vi "Get Strings from Ref.vi"(8 "error in (no error)":errorcluster, 9 "Label Prefix":string, 10 "GObj Refnum in":refnum<vi>, 11 "ArrayConstant in":refnum<class "ArrayControl.lvclass">) -> (0 "error out":errorcluster, 1 "Valid?":bool, 2 "GObj Refnum out":refnum<vi>, 3 "ArrayConstant out":refnum<class "ArrayControl.lvclass">, 4 "GObj Name":string)   [LabVIEW 2013, in "SET Project Data.lvlib" / "ArrayControl.lvclass"]
uses:
  ArrayControl.lvclass
  Control/Control.lvclass
  GObject/GObject.lvclass/GObject.ctl
  GObject/Write UID.vi
  GObject/GObject.lvclass
  SET Project Data.lvlib
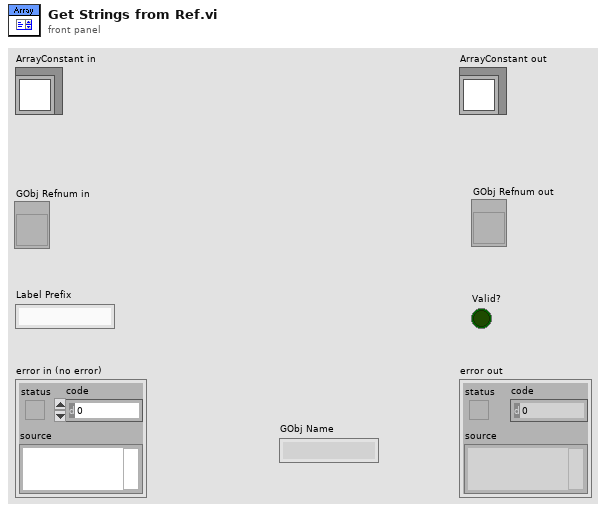
[diagram p1: front panel]
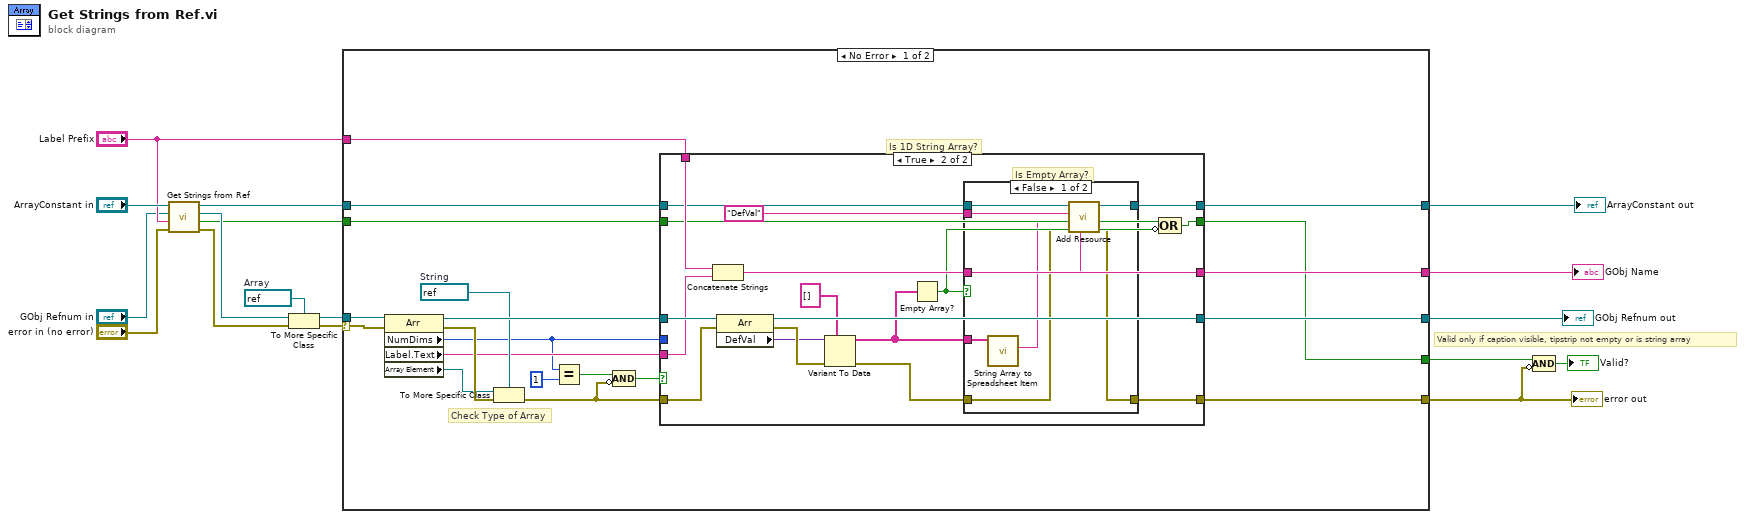
[diagram p0: block diagram]
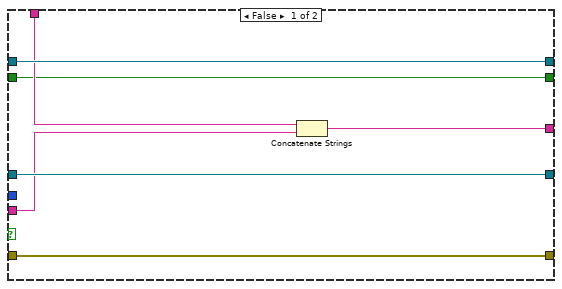
[diagram p2: hidden frame]
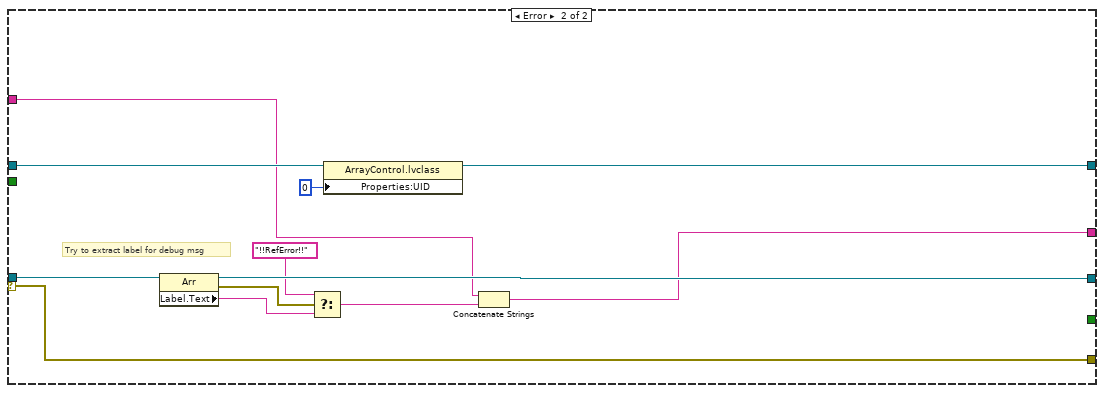
[diagram p4: hidden frame]
diagram:
  w9 = refnum<vi> refnum  # Array
  # "Valid only if caption visible, tipstrip not empty or is string array"
  n1 = call-parent "Get Strings from Ref.vi"("error in (no error)"="error in (no error)", "Label Prefix"="Label Prefix", "GObj Refnum in"="GObj Refnum in", "Control in"="ArrayConstant in") -> ("error out"=w5:errorcluster, "Valid?"=w1:bool, "GObj Refnum out"=w2:refnum<vi>, "Control out"=w7:refnum<class "ArrayControl.lvclass">)  [unwired: 3 in, 1 out]
  n2 = To More Specific Class(target class=w9, reference=w2, error in=w5) -> (specific class reference=w16:refnum<vi>, error out=w15:errorcluster)
  n3 = case shown="No Error" w15 {
    selector: w15 -> [w34 w84]
    tunnel: w16 -> [w37 w80]
    tunnel: [w32 w79] -> w12
    tunnel: [w33 w84] -> w10
    tunnel: w7 -> [w27 w83]
    tunnel: [w36 w81] -> w14
    tunnel: "Label Prefix" -> [w31 w74]
    tunnel: [w18 _] -> w17
    tunnel: [w30 w78] -> w13
    tunnel: w1 -> [w25 _]
    frame No Error {
      w28 = refnum<vi> refnum  # String
      # "Is 1D String Array?"
      # "Check Type of Array"
      n4 = property class="Arr"(reference=w37, error in=w34) -> (reference out=w35:refnum<vi>, error out=w29:errorcluster, "NumDims"=w23:u32, "Label.Text"=w24:string, "Array Element"=w26:refnum<vi>)
      n5 = To More Specific Class(target class=w28, reference=w26, error in=w29) -> (error out=w19:errorcluster)  [unwired: 1 out]
      n6 = Equal?(x=w23, y=u32 1) -> (x = y?=w21:bool)
      n7 = Compound Arithmetic op=AND(w21, invert w19) -> (w20:bool)
      n8 = case shown="True" w20 {
        tunnel: w27 -> [w44 w59]
        tunnel: [w44 w51] -> w36
        tunnel: w35 -> [w43 w62]
        tunnel: [w39 w49] -> w33
        tunnel: [w43 w61] -> w32
        tunnel: w31 -> [w42 w60]
        tunnel: [w41 w57] -> w30
        tunnel: w23 -> [_ _]
        tunnel: w25 -> [w38 w46]
        tunnel: w24 -> [w40 w52]
        tunnel: w19 -> [w39 w50]
        tunnel: [w38 w45] -> w18
        frame False {
          n9 = Concatenate Strings(w42, w40) -> (w41:string)
        }
        frame True {
          # "Is Empty Array?"
          n10 = Concatenate Strings(w60, w52) -> (w57:string)
          n11 = property class="Arr"(reference=w62, error in=w50) -> (reference out=w61:refnum<vi>, error out=w55:errorcluster, "DefVal"=w53:variant)
          n12 = Variant To Data(error in=w55, type=string[] [], Variant=w53) -> (data=w48:string[], error out=w54:errorcluster)
          n13 = Empty Array?(array=w48) -> (empty?=w47:bool)
          n14 = case shown="False" w47 {
            tunnel: w59 -> [w70 w72]
            tunnel: "DefVal" ("name") -> [w69 _]
            tunnel: w57 -> [w68 _]
            tunnel: w48 -> [w67 _]
            tunnel: w54 -> [w65 w71]
            tunnel: [w64 w72] -> w51
            tunnel: [w63 w71] -> w49
            frame False {
              n15 = call "String Array to Spreadsheet Item.vi"("Strings [] (ASCII)"=w67) -> ("Spreadsheet Item (ASCII)"=w66:string)  [unwired: 10 in]
              n16 = call "Add Resource.vi"("TagPrefix"=w68, "error in (no error)"=w65, "ItemText"=w66, "ItemName"=w69, "GObject in"=w70) -> ("error out"=w63:errorcluster, "GObject out"=w64:refnum<class "ArrayControl.lvclass">)  [unwired: 5 in]
            }
            frame True {
            }
          }
          n17 = Compound Arithmetic op=OR(w46, invert w47) -> (w45:bool)
        }
      }
    }
    frame Error {
      # "Try to extract label for debug msg"
      n18 = property class="Arr"(reference=w80) -> (reference out=w79:refnum<vi>, error out=w77:errorcluster, "Label.Text"=w75:string)  [unwired: 1 in]
      n19 = Select(t="!!RefError!!" ("Label.Text"), s=w77, f=w75) -> (s? t:f=w73:string)
      n20 = property class="ArrayControl.lvclass"(reference=w83, "Properties:UID"=0 ("UID")) -> (reference out=w81:refnum<class "ArrayControl.lvclass">)  [unwired: 1 in, 1 out]
      n21 = Concatenate Strings(w74, w73) -> (w78:string)
    }
  }
  "error out" <- w10
  "ArrayConstant out" <- w14
  "GObj Refnum out" <- w12
  "GObj Name" <- w13
  n22 = Compound Arithmetic op=AND(w17, invert w10) -> (→"Valid?":bool)
